vi "Read (Single Response).vi"(8 "error in (no error)":errorcluster, 11 "VISA resource name":refnum<visa-resource-name>) -> (0 "error out":errorcluster, 1 "Response Bundle":T1, 2 "Response":string, 3 "VISA resource name out":refnum<visa-resource-name>)   [LabVIEW 2018, in "Zaber A Series.lvlib"]
doc: "Reads a single response from the Serial buffer. The complete string is returned on the Response output, and the details of the format of the response are described here: http://www.zaber.com/wiki/Manuals/ASCII_Protocol_Manual#Replies. This VI also validates checksums if present, combines multi-packet messages if needed, parses the message, bundles the components, and returns the bundle on the Response Bundle pin. \n\nThe Response Bundle is designed to extract data from Replies only. Info and Alert type responses will not make sense in the Bundle and should be read with just the Response output. By default the only Info or Alert type responses you can expect directly follow 'help' commands. \n\nThis VI requires that the Initialize VI has been called with the same serial port. \n\nThe Data string of the response is checked for rejection responses and if any are detected will send a warning or error on the error out. The possible warnings and errors are:\n\n-1074000003 - BADCHECKSUM - The checksum of a reply message indicates a transmission error.\n-1074000004 - BADFLAGS - The reply flags field of a response was not one of the legal values.\n-1074000005 - BADPACKET - A message did not start with one of the legal marger characters.\n-1074000006 - BADSEQUENCE - A multi-packet message could not be combined.\n1073481729 - BADCHECKSUM - The checksum provided in the command message was incorrect.\n1073481730 - BADCOMMAND - The command or setting is incorrect or invalid.\n1073481731 - BADDATA - The data provided in the command is incorrect or out of range.\n1073481732 - STATUSBUSY - The device cannot be parked, nor can certain settings be changed, because it is currently busy.\n1073481733 - DEVICEONLY - An axis number was specified when trying to execute a device only command.\n1073481734 - PARKED - The device cannot move because it is currently parked.\n1073481735 - AGAIN - The stream queue is full. The command should be resent until AGAIN is not received. \n1073481736 - BADMESSAGEID - A message ID was provided, but was not either -- or a number from 0 to 99.\n1073481737 - BADAXIS - The command was sent with an axis number greater than the number of axes available.\n1073481738 - LOCKSTEP - An axis cannot be moved using normal motion commands because it is part of a lockstep group. You must use lockstep commands for motion or disable the lockstep group first.\n1073481739 - FULL - The device has run out of permanent storage and cannot accept the command. Occurs when storing to a stream buffer or when saving commands to joystick keys.\n1073481740 - NOACCESS - The command or setting is not available at the current access level.\n\nNote: This VI is set to read 100 bytes at a time, but will terminate each read when it sees the new line character in order to return only one response. It's assumed that responses will be shorter than 100 characters. If your responses exceed this for any reason, adjust the constant to a higher number."
uses:
  Zaber A Series.lvlib
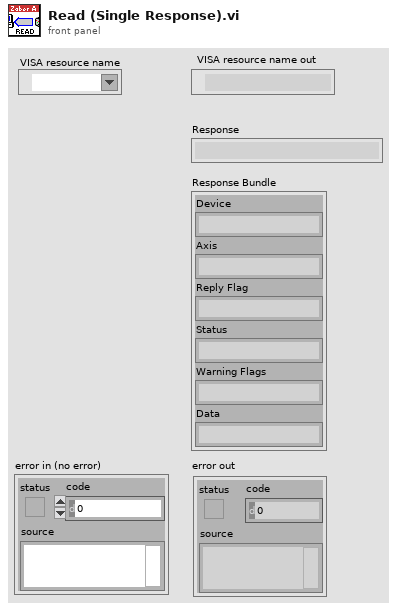
[diagram p1: front panel]
types:
  T1 = cluster{"Device":string, "Axis":string, "Reply Flag":string, "Status":string, "Warning Flags":string, "Data":string}
  T2 = cluster{string, string, string, string, string, "spreadsheet string":string}
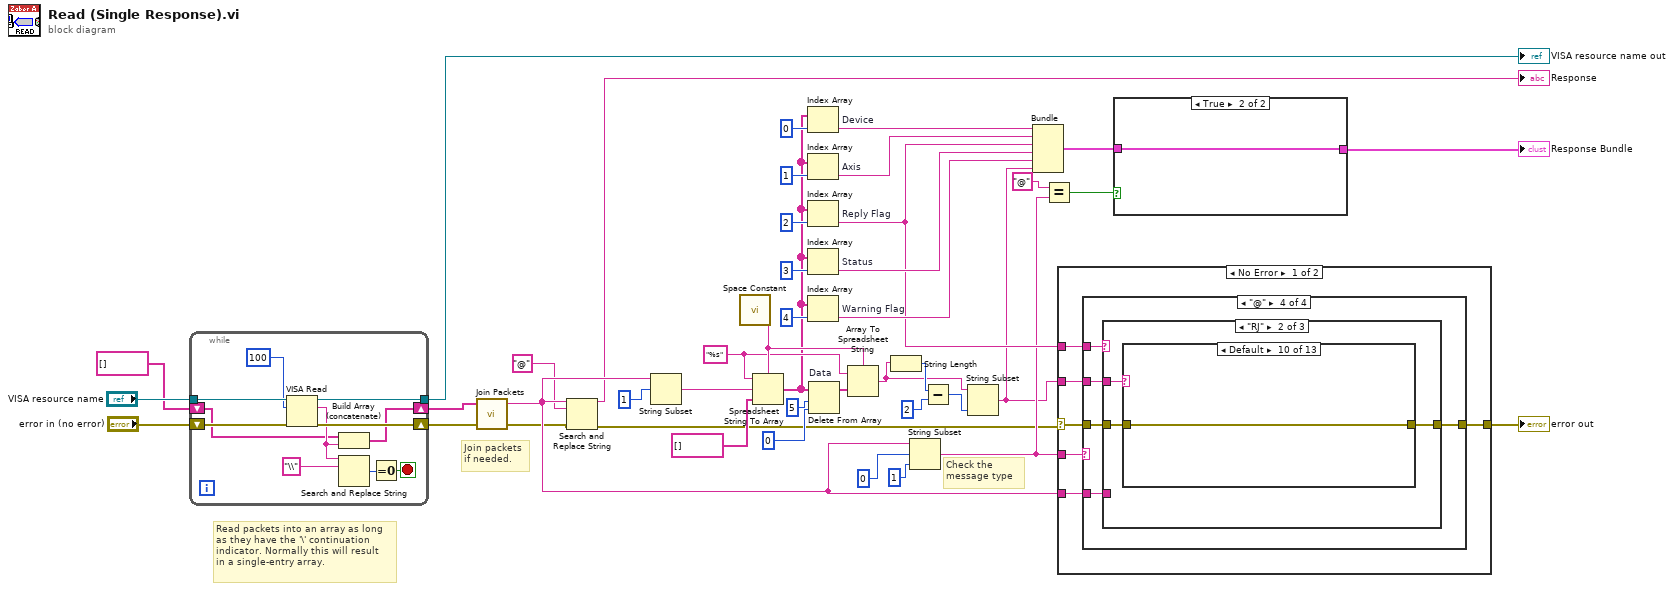
[diagram p0: block diagram]
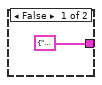
[diagram p2: hidden frame]
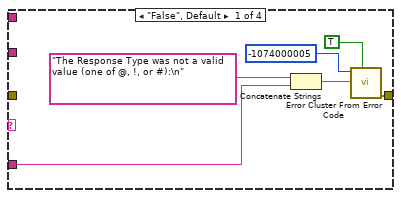
[diagram p3: hidden frame]
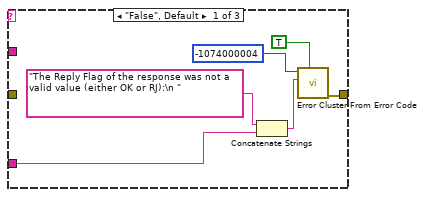
[diagram p6: hidden frame]
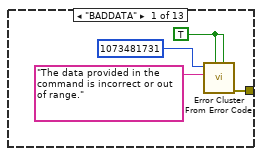
[diagram p7: hidden frame]
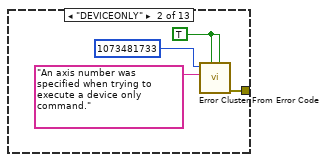
[diagram p8: hidden frame]
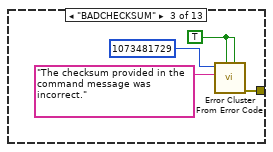
[diagram p9: hidden frame]
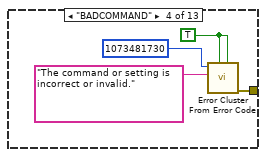
[diagram p10: hidden frame]
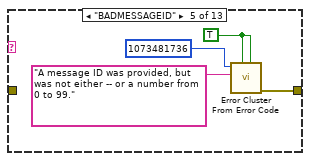
[diagram p11: hidden frame]
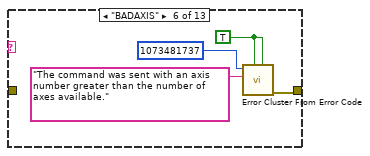
[diagram p12: hidden frame]
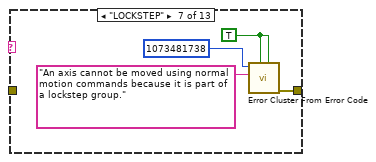
[diagram p13: hidden frame]
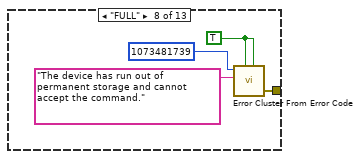
[diagram p14: hidden frame]
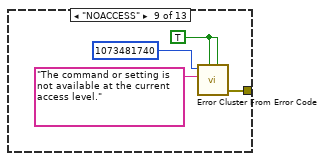
[diagram p15: hidden frame]
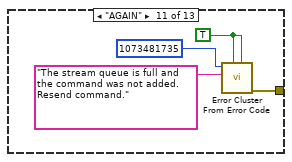
[diagram p16: hidden frame]
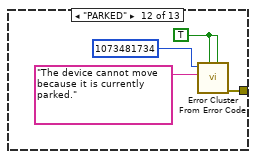
[diagram p17: hidden frame]
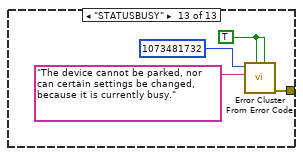
[diagram p18: hidden frame]
diagram:
  w25 = "%s" ("format string")
  # "Join packets\nif needed."
  # "Read packets into an array as long\nas they have the '\\' continuation\nindicator. Normally this will result\nin a single-entry array."
  # "Check the\nmessage type"
  n1 = while {
    shift-right: [w50] -> w6
    shift-left: "error in (no error)" -> [w53]
    shift-right: [w45] -> w7
    shift-left: string[] [] -> [w44]
    tunnel: "VISA resource name" -> [w54]
    tunnel: [w51] -> w41
    stop <- w47 stop-if-true
    n2 = VISA Read(VISA resource name=w54, byte count=u32 100, error in (no error)=w53) -> (VISA resource name out=w51:refnum<visa-resource-name>, read buffer=w46:string, error out=w50:errorcluster)  [unwired: 1 out]
    n3 = Build Array (concatenate)(w44, w46) -> (w45:string[])
    n4 = Search and Replace String(input string=w46, search string="\\") -> (number of replacements=w49:i32)  [unwired: 6 in, 3 out]
    n5 = Equal To 0?(x=w49) -> (x = 0?=w47:bool)
  }
  "VISA resource name out" <- w41
  n6 = call "Join Packets.vi"("error in (no error)"=w6, "Packets"=w7) -> ("error out"=w3:errorcluster, "Response"=w5:string)  [unwired: 2 in]
  n7 = Search and Replace String(input string=w5, search string="@" ("substring (\"\")"), error in=w3) -> (result string=→"Response":string, error out=w2:errorcluster)  [unwired: 5 in, 2 out]
  n8 = String Subset(string=w5, offset (0)=1) -> (substring=w8:string)  [unwired: 1 in]
  n9 = call <vilib>:"Space Constant.vi"() -> ("String"=w33:string)
  n10 = Spreadsheet String To Array(delimiter (Tab)=w33, format string=w25, spreadsheet string=w8, array type (2D Dbl)=string[] []) -> (array=w24:string[])
  n11 = Index Array "Device"(array=w24, index=0) -> (element=w38:string)
  n12 = Index Array "Axis"(array=w24, index=1) -> (element=w37:string)
  n13 = Index Array "Reply Flag"(array=w24, index=2) -> (element=w21:string)
  n14 = Index Array "Status"(array=w24, index=3) -> (element=w36:string)
  n15 = Index Array "Warning Flag"(array=w24, index=4) -> (element=w35:string)
  n16 = Delete From Array "Data"(array=w24, length=5, index=0) -> (array with subset deleted=w34:string[])  [unwired: 1 out]
  n17 = Array To Spreadsheet String(delimiter (Tab)=w33, array=w34, 3:w25) -> (spreadsheet string=w12:string)
  n18 = String Length(string=w12) -> (length=w14:i32)
  n19 = String Subset(string=w5, offset (0)=0, length (rest)=1 ("length (rest)")) -> (substring=w18:string)
  n20 = Subtract(x=w14, y=2) -> (x-y=w13:i32)
  n21 = String Subset(string=w12, length (rest)=w13) -> (substring=w11:string)  [unwired: 1 in]
  n22 = Bundle(w38, w37, w21, w36, w35, "spreadsheet string"=w11) -> (w20:T2)  [unwired: 1 in]
  n23 = Equal?(x="@", y=w18) -> (x = y?=w16:bool)
  n24 = case shown="No Error" w2 {
    selector: w2 -> [w58 w133]
    tunnel: [w60 w133] -> w40
    tunnel: w11 -> [w59 _]
    tunnel: w18 -> [w57 _]
    tunnel: w21 -> [w56 _]
    tunnel: w5 -> [w55 _]
    frame No Error {
      n25 = case shown="\"@\"" w57 {
        tunnel: [w64 w67 w68 w73] -> w60
        tunnel: w59 -> [_ _ _ w72]
        tunnel: w58 -> [_ w67 w68 w71]
        tunnel: w56 -> [_ _ _ w70]
        tunnel: w55 -> [w61 _ _ w69]
        frame "False", Default {
          n26 = Concatenate Strings("The Response Type was not a valid value (one of @, !, or #):\n" ("error message (\"\")"), w61) -> (w63:string)
          n27 = call <vilib>:"Error Cluster From Error Code.vi"("show call chain? (False)"=TRUE, "error message (\"\")"=w63, "error code (0)"=-1074000005) -> ("error out"=w64:errorcluster)  [unwired: 6 in]
        }
        frame "!" {
        }
        frame "#" {
        }
        frame "@" {
          n28 = case shown="\"RJ\"" w70 {
            tunnel: [w77 w82 w132] -> w73
            tunnel: w72 -> [_ w81 _]
            tunnel: w71 -> [_ w80 w132]
            tunnel: w69 -> [w76 _ _]
            frame "False", Default {
              n29 = Concatenate Strings("The Reply Flag of the response was not a valid value (either OK or RJ):\n " ("error message (\"\")"), w76) -> (w74:string)
              n30 = call <vilib>:"Error Cluster From Error Code.vi"("show call chain? (False)"=TRUE, "error message (\"\")"=w74, "error code (0)"=-1074000004) -> ("error out"=w77:errorcluster)  [unwired: 6 in]
            }
            frame "RJ" {
              n31 = case shown="Default" w81 {
                tunnel: [w83 w89 w91 w95 w99 w103 w107 w111 w115 w119 w120 w125 w129] -> w82
                tunnel: w80 -> [_ _ _ _ _ _ _ _ _ w119 _ _ _]
                frame "BADDATA" {
                  w86 = TRUE
                  n32 = call <vilib>:"Error Cluster From Error Code.vi"("is warning? (False)"=w86, "show call chain? (False)"=w86, "error message (\"\")"="The data provided in the command is incorrect or out of range." ("error message (\"\")"), "error code (0)"=1073481731) -> ("error out"=w83:errorcluster)  [unwired: 5 in]
                }
                frame "DEVICEONLY" {
                  w90 = TRUE
                  n33 = call <vilib>:"Error Cluster From Error Code.vi"("is warning? (False)"=w90, "show call chain? (False)"=w90, "error message (\"\")"="An axis number was specified when trying to execute a device only command." ("error message (\"\")"), "error code (0)"=1073481733) -> ("error out"=w89:errorcluster)  [unwired: 5 in]
                }
                frame "BADCHECKSUM" {
                  w94 = TRUE
                  n34 = call <vilib>:"Error Cluster From Error Code.vi"("is warning? (False)"=w94, "show call chain? (False)"=w94, "error message (\"\")"="The checksum provided in the command message was incorrect." ("error message (\"\")"), "error code (0)"=1073481729) -> ("error out"=w91:errorcluster)  [unwired: 5 in]
                }
                frame "BADCOMMAND" {
                  w98 = TRUE
                  n35 = call <vilib>:"Error Cluster From Error Code.vi"("is warning? (False)"=w98, "show call chain? (False)"=w98, "error message (\"\")"="The command or setting is incorrect or invalid." ("error message (\"\")"), "error code (0)"=1073481730) -> ("error out"=w95:errorcluster)  [unwired: 5 in]
                }
                frame "BADMESSAGEID" {
                  w102 = TRUE
                  n36 = call <vilib>:"Error Cluster From Error Code.vi"("is warning? (False)"=w102, "show call chain? (False)"=w102, "error message (\"\")"="A message ID was provided, but was not either -- or a number from 0 to 99." ("error message (\"\")"), "error code (0)"=1073481736) -> ("error out"=w99:errorcluster)  [unwired: 5 in]
                }
                frame "BADAXIS" {
                  w104 = TRUE
                  n37 = call <vilib>:"Error Cluster From Error Code.vi"("is warning? (False)"=w104, "show call chain? (False)"=w104, "error message (\"\")"="The command was sent with an axis number greater than the number of axes available." ("error message (\"\")"), "error code (0)"=1073481737) -> ("error out"=w103:errorcluster)  [unwired: 5 in]
                }
                frame "LOCKSTEP" {
                  w110 = TRUE
                  n38 = call <vilib>:"Error Cluster From Error Code.vi"("is warning? (False)"=w110, "show call chain? (False)"=w110, "error message (\"\")"="An axis cannot be moved using normal motion commands because it is part of a lockstep group." ("error message (\"\")"), "error code (0)"=1073481738) -> ("error out"=w107:errorcluster)  [unwired: 5 in]
                }
                frame "FULL" {
                  w112 = TRUE
                  n39 = call <vilib>:"Error Cluster From Error Code.vi"("is warning? (False)"=w112, "show call chain? (False)"=w112, "error message (\"\")"="The device has run out of permanent storage and cannot accept the command." ("error message (\"\")"), "error code (0)"=1073481739) -> ("error out"=w111:errorcluster)  [unwired: 5 in]
                }
                frame "NOACCESS" {
                  w118 = TRUE
                  n40 = call <vilib>:"Error Cluster From Error Code.vi"("is warning? (False)"=w118, "show call chain? (False)"=w118, "error message (\"\")"="The command or setting is not available at the current access level." ("error message (\"\")"), "error code (0)"=1073481740) -> ("error out"=w115:errorcluster)  [unwired: 5 in]
                }
                frame Default {
                }
                frame "AGAIN" {
                  w123 = TRUE
                  n41 = call <vilib>:"Error Cluster From Error Code.vi"("is warning? (False)"=w123, "show call chain? (False)"=w123, "error message (\"\")"="The stream queue is full and the command was not added. Resend command." ("error message (\"\")"), "error code (0)"=1073481735) -> ("error out"=w120:errorcluster)  [unwired: 5 in]
                }
                frame "PARKED" {
                  w127 = TRUE
                  n42 = call <vilib>:"Error Cluster From Error Code.vi"("is warning? (False)"=w127, "show call chain? (False)"=w127, "error message (\"\")"="The device cannot move because it is currently parked." ("error message (\"\")"), "error code (0)"=1073481734) -> ("error out"=w125:errorcluster)  [unwired: 5 in]
                }
                frame "STATUSBUSY" {
                  w131 = TRUE
                  n43 = call <vilib>:"Error Cluster From Error Code.vi"("is warning? (False)"=w131, "show call chain? (False)"=w131, "error message (\"\")"="The device cannot be parked, nor can certain settings be changed, because it is currently busy." ("error message (\"\")"), "error code (0)"=1073481732) -> ("error out"=w129:errorcluster)  [unwired: 5 in]
                }
              }
            }
            frame "OK" {
            }
          }
        }
      }
    }
    frame Error {
    }
  }
  "error out" <- w40
  n44 = case shown="True" w16 {
    tunnel: w20 -> [_ w135]
    tunnel: [T2 {"", "", "", "", "", "spreadsheet string"=""} ("output cluster") w135] -> w19
    frame False {
    }
    frame True {
    }
  }
  "Response Bundle" <- w19
